vi "Get Sound Samples.vi"(0 "error in":errorcluster, 1 "task ID":T2 format="%.0x", 2 "sound file refnum":T1, 3 "Sample Start Position":i32, 4 "Samples Per Read":i32) -> (5 "end of file?":bool, 7 "error out":errorcluster, 9 "data":waveform(dbl)[](array[waveform]), 10 "Next Sample Start Position":i32)   [LabVIEW 2015, in "LabVIEW Interface for Arduino.lvlib"]
uses:
  <vilib>/LabVIEW Interface for Arduino/LabVIEW Interface for Arduino.lvlib
  <vilib>/sound2/lvsound2.llb/Sound Output Task ID.ctl
  <vilib>/sound2/lvsound2.llb/Sound File Refnum.ctl
  <vilib>/sound2/lvsound2.llb/Sound File Position.ctl
  <vilib>/sound2/lvsound2.llb/Sound File Read (DBL).vi
  <vilib>/sound2/lvsound2.llb/Sound Output Write (DBL).vi
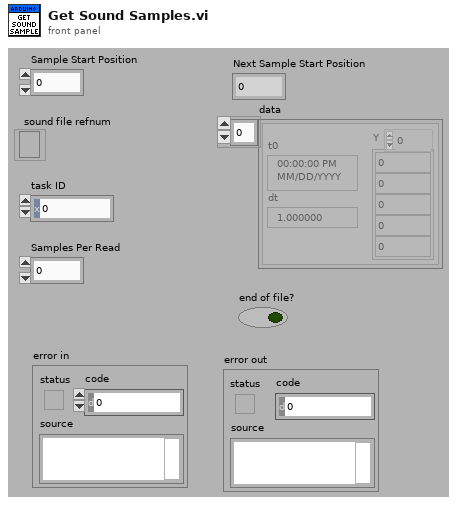
[diagram p1: front panel]
types:
  T1 = typedef "Sound File Refnum.ctl" = refnum<file>
  T2 = typedef "Sound Output Task ID.ctl" = u32
  T3 = typedef "Sound File Position.ctl" = u16
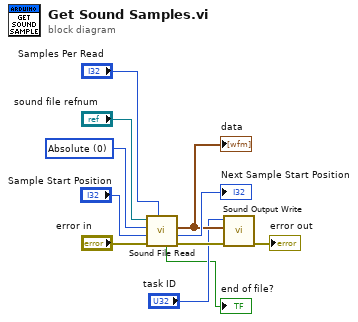
[diagram p0: block diagram]
diagram:
  w3 = T3 0 items=["Absolute"=0, "Relative"=2] ("position mode")
  n1 = call-poly <vilib>:"Sound File Read.vi"("number of samples/ch (-1: all)"="Samples Per Read", "error in (no error)"="error in", "position offset"="Sample Start Position", "position mode"=w3, "sound file refnum"="sound file refnum") -> ("error out"=w6:errorcluster, "offset"=→"Next Sample Start Position":i32, "data"=w8:waveform(dbl)[], "end of file?"=→"end of file?":bool)  [unwired: 2 in, 1 out]
  "data" <- w8
  n2 = call-poly <vilib>:"Sound Output Write.vi"("error in (no error)"=w6, "data"=w8, "task ID"="task ID") -> ("error out"=→"error out":errorcluster)  [unwired: 7 in, 1 out]
